vi "LoadGlobalConfigure.vi"(8 "error in (no error)":errorcluster caption="error in", 11 "ReadExcel？":bool) -> (0 "error out":errorcluster, 2 "AngleParams":T1, 3 "ConfigParams":T2)   [LabVIEW 2024]
uses:
  Ctrls/GlobalConfigure.ctl
  Ctrls/AngleVerify.ctl
  <vilib>/Utility/config.llb/Read Key (String).vi
  <vilib>/Utility/config.llb/NI_LVConfig.lvlib
panel:
  out "date string":string
  # "上位机传递 参数至TestStand  的全局变量   文件路径"
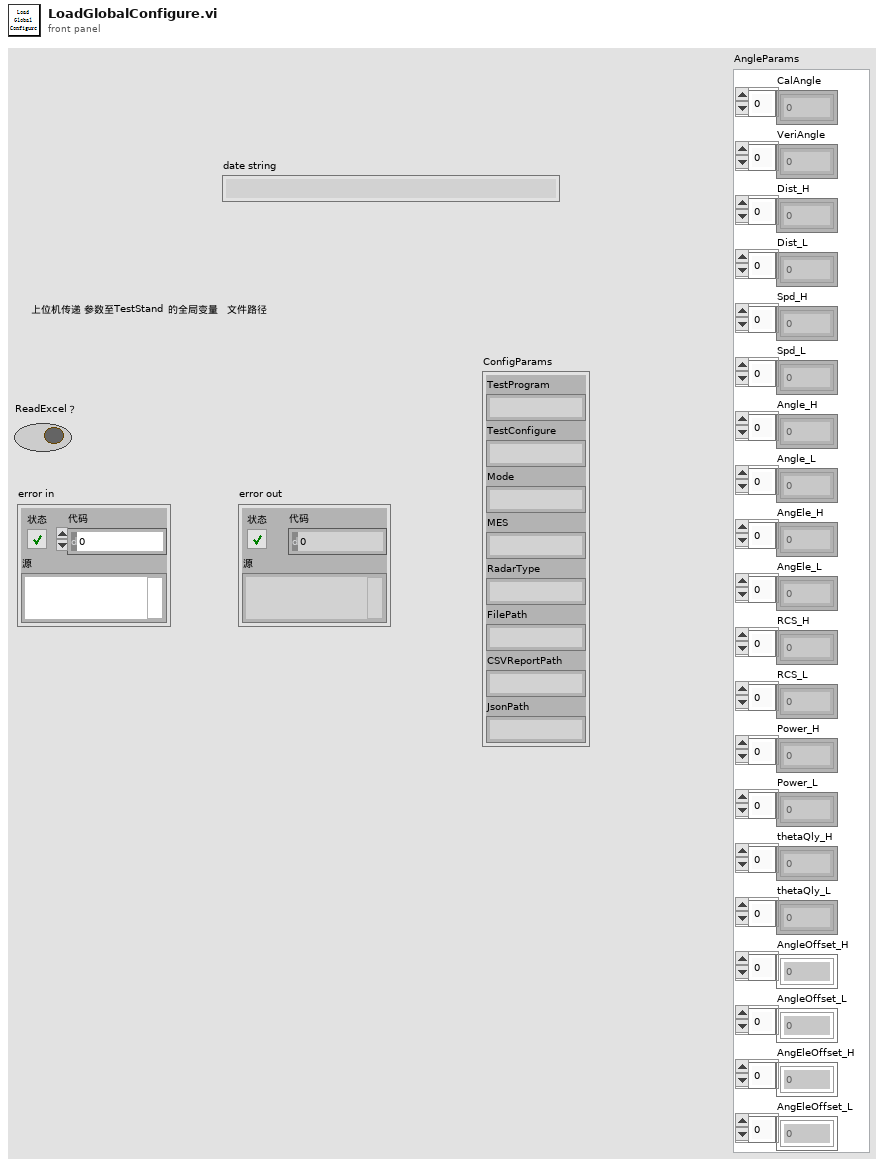
[diagram p1: front panel]
types:
  T1 = typedef "AngleVerify.ctl" = cluster{"CalAngle":dbl[], "VeriAngle":dbl[], "Dist_H":dbl[], "Dist_L":dbl[], "Spd_H":dbl[], "Spd_L":dbl[], "Angle_H":dbl[], "Angle_L":dbl[], "AngEle_H":dbl[], "AngEle_L":dbl[], "RCS_H":dbl[], "RCS_L":dbl[], "Power_H":dbl[], "Power_L":dbl[], "thetaQly_H":dbl[], "thetaQly_L":dbl[], "AngleOffset_H":dbl[], "AngleOffset_L":dbl[], "AngEleOffset_H":dbl[], "AngEleOffset_L":dbl[]}
  T2 = typedef "GlobalConfigure.ctl" = cluster{"TestProgram":string, "TestConfigure":string, "Mode":string, "MES":string, "RadarType":string, "FilePath":string, "CSVReportPath":string, "JsonPath":string}
  T3 = typedef "NI_LVConfig.lvlib/Config Data RefNum.ctl" = refnum<k1>
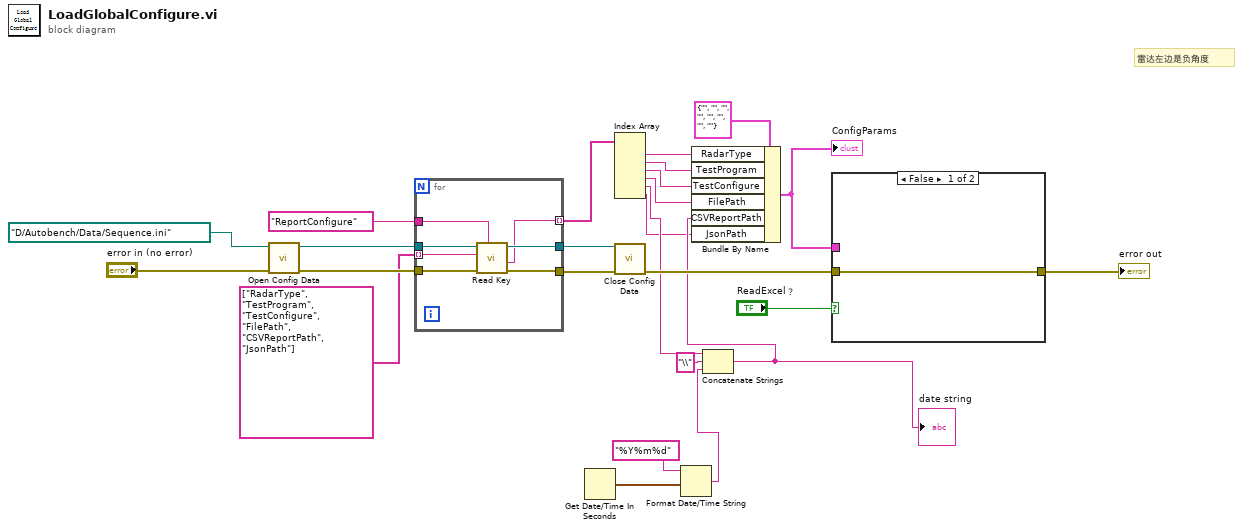
[diagram p0: block diagram]
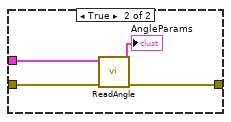
[diagram p2: hidden frame]
diagram:
  # "雷达左边是负角度"
  n1 = call <vilib>:"Open Config Data.vi"("error in (no error)"="error in (no error)", "configuration file path"=path "D:/Autobench/Data/Sequence.ini") -> ("error out"=w22:errorcluster, "refnum"=w21:T3)  [unwired: 7 in, 1 out]
  n2 = for {
    tunnel: w22 -> [w31]
    tunnel: w21 -> [w32]
    tunnel: [w30] -> w25
    tunnel: [w29] -> w24
    tunnel: "ReportConfigure" ("section") -> [w28]
    tunnel: [w27] -> w17 mode=indexing
    tunnel: string[] ["RadarType", "TestProgram", "TestConfigure", "FilePath", "CSVReportPath", "JsonPath"] -> [w26] mode=indexing
    n3 = call-poly <vilib>:"Read Key.vi"("section"=w28, "error in (no error)"=w31, "key"=w26, "refnum"=w32) -> ("error out"=w29:errorcluster, "value"=w27:string, "refnum out"=w30:T3)  [unwired: 4 in, 1 out]
  }
  n4 = Get Date/Time In Seconds() -> (seconds since 1Jan1904=w7:timestamp)
  n5 = Index Array(array=w17) -> (element #1=w16:string, element #2=w15:string, element #3=w14:string, element #4=w12:string, element #5=w5:string, element #6=w1:string)  [unwired: 6 in]
  n6 = call <vilib>:"Close Config Data.vi"("error in (no error)"=w24, "refnum"=w25) -> ("error out"=w10:errorcluster)  [unwired: 8 in, 1 out]
  n7 = Format Date/Time String(time format string (%c)="%Y%m%d", seconds (now)=w7) -> (date/time string=w3:string)  [unwired: 1 in]
  n8 = Concatenate Strings(w5, "\\" ("string"), w3) -> (w2:string)
  "date string" <- w2
  n9 = Bundle By Name(cluster=T2 {"TestProgram"="", "TestConfigure"="", "Mode"="", "MES"="", "RadarType"="", "FilePath"="", "CSVReportPath"="", "JsonPath"=""}, "RadarType"=w16, "TestProgram"=w15, "TestConfigure"=w14, "FilePath"=w12, "CSVReportPath"=w2, "JsonPath"=w1) -> (w11:T2)
  "ConfigParams" <- w11
  n10 = case shown="False" "ReadExcel？" {
    tunnel: w11 -> [_ w37]
    tunnel: w10 -> [w33 w36]
    tunnel: [w33 w35] -> w9
    frame False {
    }
    frame True {
      n11 = call "ReadAngle.vi"("error in (no error)"=w36, "ConfigParams"=w37) -> ("error out"=w35:errorcluster, "Cluster"=→"AngleParams":T1)  [unwired: 8 in]
    }
  }
  "error out" <- w9
